vi "RTI DDS_Copy.vi"(0 "XRef":T5, 1 "State In":T1) -> (14 "Reply":T3, 15 "Fatal Error Out":T2, 16 "State Out":T1)   [LabVIEW 2020, in "RTI DDS.xnode"]
doc: "Download the RTI DDS Toolkit for LabVIEW."
uses:
  <vilib>/RTI DDS Toolkit/_RTI DDS XNode/RTI DDS.xnode
  <vilib>/XNodeSupport/XNodeString.ctl
  <vilib>/XNodeSupport/NI_XNodeSupport.lvlib
  <vilib>/XNodeSupport/XNodeStringArray.ctl
  <vilib>/XNodeSupport/XNodeXNodeRef.ctl
  <vilib>/XNodeSupport/XNodeErrorCluster.ctl
  <vilib>/RTI DDS Toolkit/_RTI DDS XNode/RTI DDS.ctl
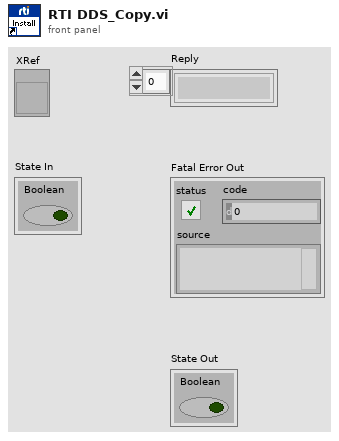
[diagram p1: front panel]
types:
  T1 = typedef "RTI DDS.xnode/RTI DDS.ctl" = cluster{"Boolean":bool}
  T2 = typedef "NI_XNodeSupport.lvlib/XNodeErrorCluster.ctl" = errorcluster
  T3 = typedef "NI_XNodeSupport.lvlib/XNodeStringArray.ctl" = T4[]
  T4 = typedef "NI_XNodeSupport.lvlib/XNodeString.ctl" = string
  T5 = typedef "NI_XNodeSupport.lvlib/XNodeXNodeRef.ctl" = refnum<vi>
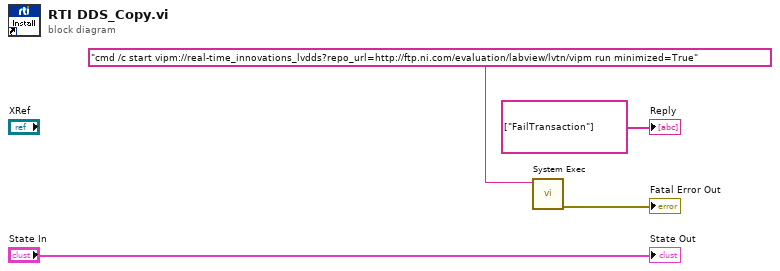
[diagram p0: block diagram]
diagram:
  n1 = call <vilib>:"System Exec.vi"("command line"="cmd /c start vipm://real-time_innovations_lvdds?repo_url=http://ftp.ni.com/evaluation/labview/lvtn/vipm run minimized=True" ("URL")) -> ("error out"=→"Fatal Error Out":errorcluster)  [unwired: 7 in, 3 out]
  "Reply" <- T3 ["FailTransaction"] ("Reply")
  "State Out" <- "State In"
